vi "Read OTP Values from ini file.vi"(8 "error in (no error)":errorcluster, 10 "configuration file path":path, 11 "Test Framework.lvclass":refnum<class "Test Framework.lvclass">) -> (0 "error out":errorcluster, 2 "OTP Cluster Out":T1, 3 "Test Framework.lvclass out":refnum<class "Test Framework.lvclass">)   [LabVIEW 2020, in "Test Framework.lvclass"]
uses:
  Test Framework/Test Framework.lvclass
  Measurements/Controls/OTP_Cluster.ctl
  Test Framework/Test Framework.lvclass/Test Framework.ctl
  <vilib>/Utility/config.llb/Read Key (String).vi
  <vilib>/Utility/config.llb/Read Key (Double).vi
  <vilib>/Utility/config.llb/Read Key (I32).vi
  <vilib>/Utility/config.llb/Read Key (Boolean).vi
  <vilib>/Utility/config.llb/NI_LVConfig.lvlib
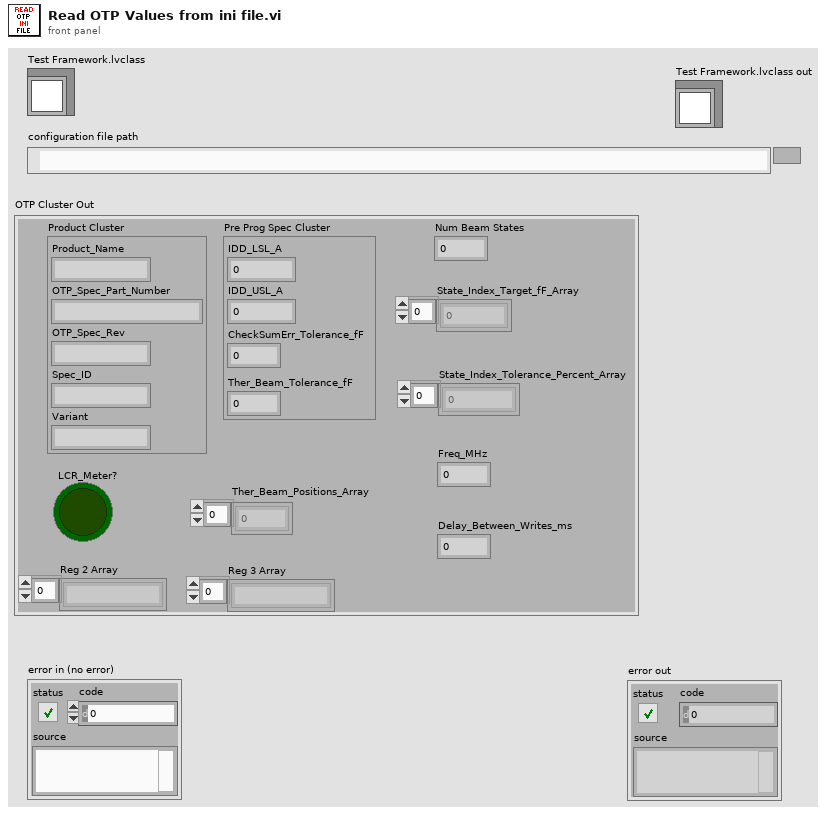
[diagram p1: front panel]
types:
  T1 = typedef "OTP_Cluster.ctl" = cluster{"Product Cluster":cluster{"Product_Name":string, "OTP_Spec_Part_Number":string, "OTP_Spec_Rev":string, "Spec_ID":string, "Variant":string}, "Pre Prog Spec Cluster":cluster{"IDD_LSL_A":dbl, "IDD_USL_A":dbl, "CheckSumErr_Tolerance_fF":dbl, "Ther_Beam_Tolerance_fF":dbl}, "LCR_Meter?":bool, "Reg 2 Array":string[], "Reg 3 Array":string[], "Num Beam States":i32, "State_Index_Target_fF_Array":dbl[], "State_Index_Tolerance_Percent_Array":dbl[], "Freq_MHz":dbl, "Delay_Between_Writes_ms":i32, "Ther_Beam_Positions_Array":i8[]}
  T2 = typedef "NI_LVConfig.lvlib/Config Data RefNum.ctl" = refnum<k1>
  T3 = cluster{"[0]":string, "[1]":string, "[2]":string, "[3]":string, "[4]":string}
  T4 = cluster{"[0]":dbl, "[1]":dbl, "[2]":dbl, "[3]":dbl}
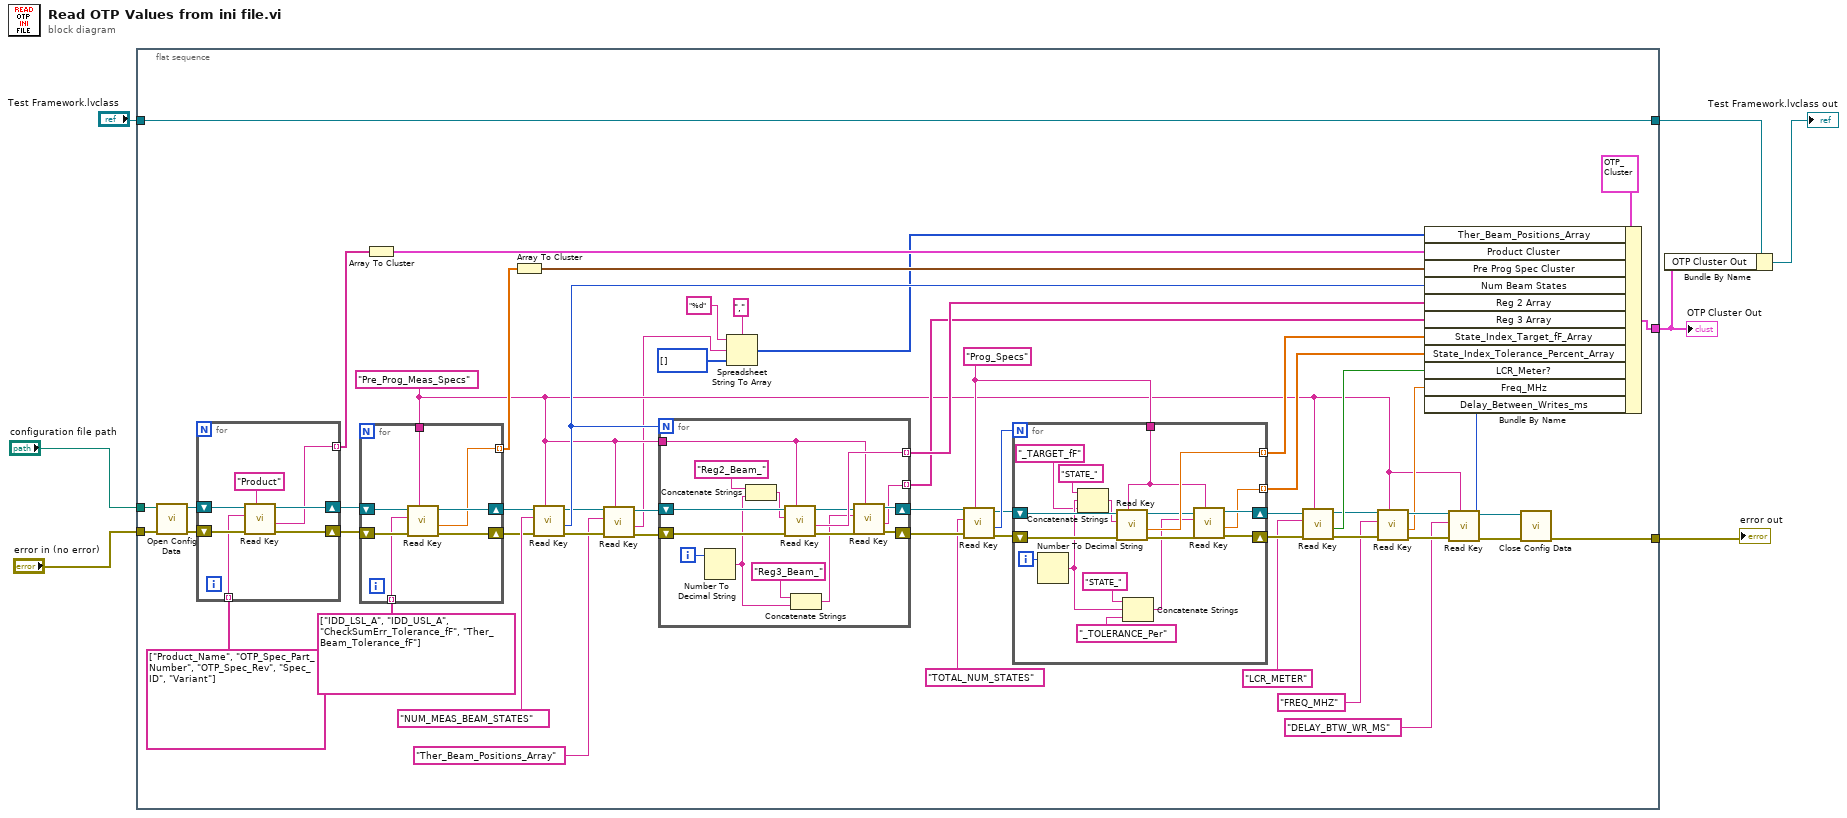
[diagram p0: block diagram]
diagram:
  n1 = flat-sequence {
    tunnel: "configuration file path" -> [w63]
    tunnel: "error in (no error)" -> [w62]
    tunnel: [w61] -> w5
    tunnel: [w38] -> w1
    tunnel: "Test Framework.lvclass" -> [w21]
    tunnel: [w21] -> w3
    frame #0 {
      w47 = "Prog_Specs" ("section")
      w14 = "Pre_Prog_Meas_Specs" ("section")
      n2 = call <vilib>:"Open Config Data.vi"("error in (no error)"=w62, "configuration file path"=w63) -> ("error out"=w58:errorcluster, "refnum"=w59:T2)  [unwired: 7 in, 1 out]
      n3 = for {
        shift-right: [w91] -> w55
        shift-left: w59 -> [w94]
        shift-right: [w92] -> w54
        shift-left: w58 -> [w93]
        tunnel: string[] ["Product_Name", "OTP_Spec_Part_Number", "OTP_Spec_Rev", "Spec_ID", "Variant"] -> [w89] mode=indexing
        tunnel: [w88] -> w56 mode=indexing
        n4 = call-poly <vilib>:"Read Key.vi"("section"="Product", "error in (no error)"=w93, "key"=w89, "refnum"=w94) -> ("error out"=w92:errorcluster, "value"=w88:string, "refnum out"=w91:T2)  [unwired: 4 in, 1 out]
      }
      n5 = for {
        shift-right: [w84] -> w52
        shift-left: w55 -> [w87]
        shift-right: [w85] -> w53
        shift-left: w54 -> [w86]
        tunnel: string[] ["IDD_LSL_A", "IDD_USL_A", "CheckSumErr_Tolerance_fF", "Ther_Beam_Tolerance_fF"] -> [w83] mode=indexing
        tunnel: [w82] -> w50 mode=indexing
        tunnel: w14 -> [w81]
        n6 = call-poly <vilib>:"Read Key.vi"("section"=w81, "error in (no error)"=w86, "key"=w83, "refnum"=w87) -> ("error out"=w85:errorcluster, "value"=w82:dbl, "refnum out"=w84:T2)  [unwired: 4 in, 1 out]
      }
      n7 = Array To Cluster(array=w56) -> (cluster=w39:T3)
      n8 = Array To Cluster(array=w50) -> (cluster=w19:T4)
      n9 = call-poly <vilib>:"Read Key.vi"("section"=w14, "error in (no error)"=w53, "key"="NUM_MEAS_BEAM_STATES", "refnum"=w52) -> ("error out"=w18:errorcluster, "value"=w37:i32, "refnum out"=w16:T2)  [unwired: 4 in, 1 out]
      n10 = call-poly <vilib>:"Read Key.vi"("section"=w14, "error in (no error)"=w18, "key"="Ther_Beam_Positions_Array", "refnum"=w16) -> ("error out"=w17:errorcluster, "value"=w8:string, "refnum out"=w15:T2)  [unwired: 4 in, 1 out]
      n11 = for {
        N: w37 -> [_]
        shift-right: [w102] -> w48
        shift-left: w15 -> [w109]
        shift-right: [w103] -> w49
        shift-left: w17 -> [w108]
        tunnel: [w105] -> w36 mode=indexing
        tunnel: w14 -> [w100]
        tunnel: [w96] -> w35 mode=indexing
        i -> [w107]
        n12 = Number To Decimal String(number=w107) -> (decimal integer string=w98:string)  [unwired: 1 in]
        n13 = Concatenate Strings("Reg2_Beam_" ("key"), w98) -> (w106:string)
        n14 = call-poly <vilib>:"Read Key.vi"("section"=w100, "error in (no error)"=w108, "key"=w106, "refnum"=w109) -> ("error out"=w104:errorcluster, "value"=w105:string, "refnum out"=w101:T2)  [unwired: 4 in, 1 out]
        n15 = Concatenate Strings("Reg3_Beam_" ("key"), w98) -> (w97:string)
        n16 = call-poly <vilib>:"Read Key.vi"("section"=w100, "error in (no error)"=w104, "key"=w97, "refnum"=w101) -> ("error out"=w103:errorcluster, "value"=w96:string, "refnum out"=w102:T2)  [unwired: 4 in, 1 out]
      }
      n17 = Spreadsheet String To Array(delimiter (Tab)=",", format string="%d", spreadsheet string=w8, array type (2D Dbl)=i8[] []) -> (array=w9:i8[])
      n18 = call-poly <vilib>:"Read Key.vi"("section"=w47, "error in (no error)"=w49, "key"="TOTAL_NUM_STATES", "refnum"=w48) -> ("error out"=w43:errorcluster, "value"=w45:i32, "refnum out"=w44:T2)  [unwired: 4 in, 1 out]
      n19 = for {
        N: w45 -> [_]
        shift-right: [w73] -> w41
        shift-left: w44 -> [w80]
        shift-right: [w74] -> w42
        shift-left: w43 -> [w79]
        tunnel: [w76] -> w34 mode=indexing
        tunnel: [w68] -> w33 mode=indexing
        tunnel: w47 -> [w65]
        i -> [w78]
        n20 = Number To Decimal String(number=w78) -> (decimal integer string=w70:string)  [unwired: 1 in]
        n21 = Concatenate Strings("STATE_" ("key"), w70, "_TARGET_fF" ("string")) -> (w77:string)
        n22 = call-poly <vilib>:"Read Key.vi"("section"=w65, "error in (no error)"=w79, "key"=w77, "refnum"=w80) -> ("error out"=w75:errorcluster, "value"=w76:dbl, "refnum out"=w72:T2)  [unwired: 4 in, 1 out]
        n23 = Concatenate Strings("STATE_" ("key"), w70, "_TOLERANCE_Per" ("string")) -> (w69:string)
        n24 = call-poly <vilib>:"Read Key.vi"("section"=w65, "error in (no error)"=w75, "key"=w69, "refnum"=w72) -> ("error out"=w74:errorcluster, "value"=w68:dbl, "refnum out"=w73:T2)  [unwired: 4 in, 1 out]
      }
      n25 = call-poly <vilib>:"Read Key.vi"("section"=w14, "error in (no error)"=w42, "key"="LCR_METER", "refnum"=w41) -> ("error out"=w31:errorcluster, "value"=w32:bool, "refnum out"=w30:T2)  [unwired: 4 in, 1 out]
      n26 = call-poly <vilib>:"Read Key.vi"("section"=w14, "error in (no error)"=w31, "key"="FREQ_MHZ", "refnum"=w30) -> ("error out"=w29:errorcluster, "value"=w23:dbl, "refnum out"=w28:T2)  [unwired: 4 in, 1 out]
      n27 = call-poly <vilib>:"Read Key.vi"("section"=w14, "error in (no error)"=w29, "key"="DELAY_BTW_WR_MS", "refnum"=w28) -> ("error out"=w26:errorcluster, "value"=w22:i32, "refnum out"=w27:T2)  [unwired: 4 in, 1 out]
      n28 = Bundle By Name(cluster=T1 {"Product Cluster"={"Product_Name"="", "OTP_Spec_Part_Number"="", "OTP_Spec_Rev"="", "Spec_ID"="", "Variant"=""}, "Pre Prog Spec Cluster"={"IDD_LSL_A"=0.0, "IDD_USL_A"=0.0, "CheckSumErr_Tolerance_fF"=0.0, "Ther_Beam_Tolerance_fF"=0.0}, "LCR_Meter?"=FALSE, "Reg 2 Array"=[], "Reg 3 Array"=[], "Num Beam States"=0, "State_Index_Target_fF_Array"=[], "State_Index_Tolerance_Percent_Array"=[], "Freq_MHz"=0.0, "Delay_Between_Writes_ms"=0, "Ther_Beam_Positions_Array"=[]} ("OTP Cluster Out"), "Ther_Beam_Positions_Array"=w9, "Product Cluster"=w39, "Pre Prog Spec Cluster"=w19, "Num Beam States"=w37, "Reg 2 Array"=w36, "Reg 3 Array"=w35, "State_Index_Target_fF_Array"=w34, "State_Index_Tolerance_Percent_Array"=w33, "LCR_Meter?"=w32, "Freq_MHz"=w23, "Delay_Between_Writes_ms"=w22) -> (w38:T1)
      n29 = call <vilib>:"Close Config Data.vi"("error in (no error)"=w26, "refnum"=w27) -> ("error out"=w61:errorcluster)  [unwired: 8 in, 1 out]
    }
  }
  n30 = Bundle By Name(cluster=w3, "OTP Cluster Out"=w1) -> (→"Test Framework.lvclass out":refnum<class "Test Framework.lvclass">)
  "error out" <- w5
  "OTP Cluster Out" <- w1
